vi "Read Transport.vi"(11 "Setup in":refnum<class "Setup.lvclass">) -> (2 "Transport":refnum<class "Transport.lvclass">)   [LabVIEW 2025, in "jettl.lvlib" / "Setup.lvlib" / "Setup.lvclass"]
uses:
  Setup.lvclass
  Transport/Transport/Transport.lvclass
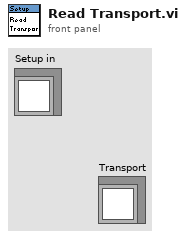
[diagram p1: front panel]
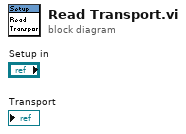
[diagram p0: block diagram]
diagram:
